vi "get_unbinned_mod.vi"() -> (0 "IntegralCount":u32, 1 "Histogram":u32[](array[numeric]))   [LabVIEW 2013]
uses:
  phlib.dll
panel:
  out "Overflow":bool
  out "Flags":i32 format="%.0b"
  in  "file refnum":refnum<file>
  out "count":i32
  out "subarray":u8[](array[numeric])
  out "dig here?":bool
  out "Counts/s":dbl format="%.2f"
  out "Data":u8[](array[numeric])
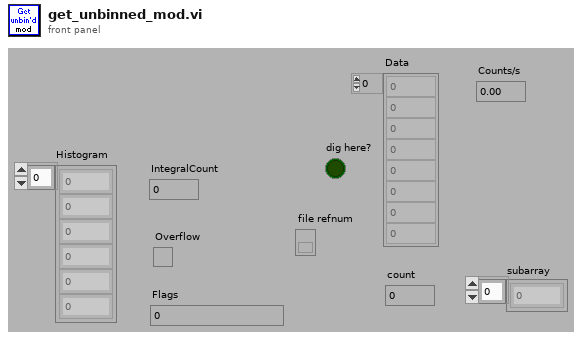
[diagram p1: front panel]
types:
  T1 = cluster{"Z_n":i32[], "devidx":i32, "initialized":bool, "acq time":i32, "Bin size":enum16{"1", "2", "4", "8", "16", "32", "64", "128"}, "# bins":i32, "sync rate":i32, "truncate":bool}
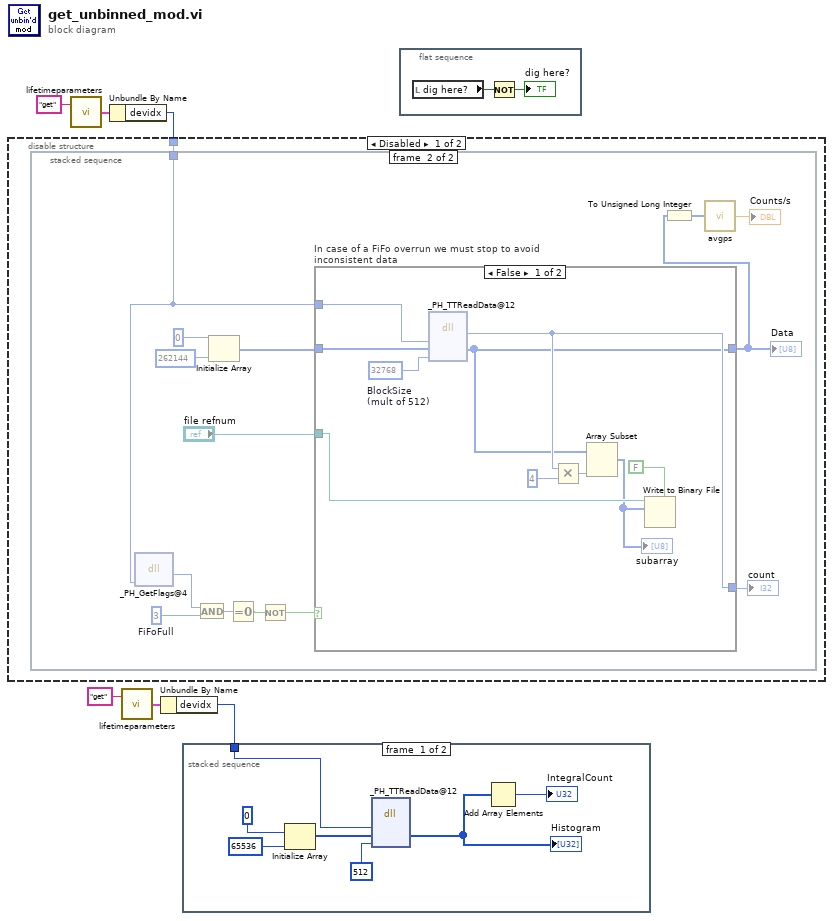
[diagram p0: block diagram]
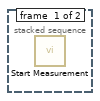
[diagram p2: hidden frame]
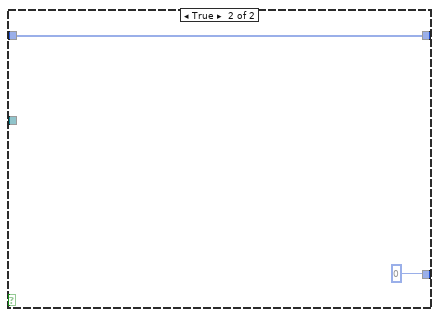
[diagram p3: hidden frame]
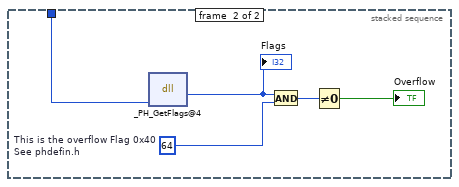
[diagram p5: hidden frame]
diagram:
  n1 = call "lifetimeparameters.vi"("command"="get") -> ("Params out"=w5:T1)  [unwired: 1 in]
  n2 = Unbundle By Name(w5) -> ("devidx"=w4:i32)
  n3 = disable-structure shown="Disabled" {
    disable-tunnel: w4 -> [w7 _]
    frame Disabled {
      n4 = stacked-sequence {
        tunnel: w7 -> [_ w11]
        frame #0 {
          n5 = call "Start Measurement.vi"() -> ()  [unwired: 1 in]
        }
        frame #1 {
          w19 = 3  # FiFoFull
          n6 = dll-call lib="phlib.dll" fn="_PH_GetFlags@4" label="PH_GetFlags"("devidx"=w11) -> (w17:i32)  [unwired: 4 in, 2 out]
          n7 = And(x=w17, y=w19) -> (x .and. y?=w18:i32)
          n8 = Initialize Array(u8 0, 262144) -> (w12:u8[])
          n9 = Equal To 0?(x=w18) -> (x = 0?=w16:bool)
          n10 = Not ("CTCDone")(x=w16) -> (.not. x?=w15:bool)
          n11 = case "In case of a FiFo overrun we must stop to avoid inconsistent data" shown="False" w15 {
            tunnel: w12 -> [w29 w33]
            tunnel: [w30 0] -> w21
            tunnel: [w28 w33] -> w8
            tunnel: "file refnum" -> [w31 _]
            tunnel: w11 -> [w26 _]
            frame False {
              w27 = 32768  # BlockSize (mult of 512)
              n12 = dll-call lib="phlib.dll" fn="_PH_TTReadData@12" label="PH_TTReadData"("devidx"=w26, "buffer"=w29, "blocksize"=w27) -> (w30:i32, "buffer"=w28:u8[])  [unwired: 5 in, 2 out]
              n13 = Multiply(x=w30, y=4) -> (x*y=w25:i32)
              n14 = Array Subset(array=w28, length=w25) -> (w22:u8[])  [unwired: 1 in]
              "subarray" <- w22
              n15 = Write to Binary File(file (use dialog)=w31, data=w22, 5:FALSE ("prepend array or string size? (T)")) -> ()  [unwired: 3 in, 3 out]
            }
            frame True {
            }
          }
          "count" <- w21
          "Data" <- w8
          n16 = To Unsigned Long Integer(number=w8) -> (unsigned 32bit integer=w10:u32[])
          n17 = call "avgps.vi"("data"=w10) -> ("Avg cts/s"=→"Counts/s":dbl)
        }
      }
    }
    frame Enabled {
    }
  }
  n18 = call "lifetimeparameters.vi"("command"="get") -> ("Params out"=w2:T1)  [unwired: 1 in]
  n19 = Unbundle By Name(w2) -> ("devidx"=w1:i32)
  n20 = stacked-sequence {
    tunnel: w1 -> [w35 w41]
    frame #0 {
      n21 = Initialize Array "Initialize Array"(u8 0, 65536) -> (w37:u8[])
      n22 = dll-call lib="phlib.dll" fn="_PH_TTReadData@12" label="PH_TTReadData"("devidx"=w35, "buffer"=w37, "block"=512) -> ("buffer"=w34:u8[])  [unwired: 6 in, 2 out]
      "Histogram" <- w34
      n23 = Add Array Elements(numeric array=w34) -> (sum=→"IntegralCount":u8)
    }
    frame #1 {
      w45 = 64  # This is the overflow Flag 0x40 See phdefin.h
      n24 = dll-call lib="phlib.dll" fn="_PH_GetFlags@4" label="PH_GetFlags"("devidx"=w41) -> (w44:i32)  [unwired: 4 in, 2 out]
      "Flags" <- w44
      n25 = And(x=w44, y=w45) -> (x .and. y?=w42:i32)
      n26 = Not Equal To 0?(x=w42) -> (x != 0?=→"Overflow":bool)
    }
  }
  n27 = flat-sequence {
    frame #0 {
      n28 = local read "dig here?"() -> (w46:bool)
      n29 = Not(x=w46) -> (.not. x?=→"dig here?":bool)
    }
  }
